vi "Open Follower Falcon.vi"(6 "Supply Current Limit Configuration":T1, 7 "refnum name":string="TalonSRX", 8 "error in (no error)":errorcluster, 9 "Master Controller to Follow":T2={"DeviceStatus"={"status"=FALSE, "code"=0, "source"=""}, "Type"=enum."PWM", "PWM"={"PWM Channel"=enum."PWM 1", "DeadBand"={"Name"="", "maxPositivePwm"=0, "minPositivePwm"=0, "centerPwm"=0, "maxNegativePwm"=0, "minNegativePwm"=0, "angularRange"=0}}, "CAN"={"Device Number"=255, "SetOutput VI Ref"=variant(enum8{"Percent VBus", "Current", "Speed", "Position", "Voltage"} enum."Percent VBus"), "GetOutput VI Ref"=variant(refnum<k1> refnum), "Enable VI Ref"=variant(dbl 12.0), "Disable VI Ref"=variant(enum8{"Percent VBus", "Speed", "Position", "Slave", "Unchanged / Invalid", "Voltage Compensation", "Current", "Motion Profile"} enum."Percent VBus"), "Data"=variant}, "Invert"=FALSE, "DIO PWM"={"PWM \"Enable\" Channel"=enum."Invalid", "DIOChannel"=enum."Invalid", "PWM Rate"=0.0}}, 10 "Invert?":bool, 11 "Device Number":u8) -> (0 "error out":errorcluster)   [LabVIEW 2019, in "Drive.lvlib" / "Falcon500.lvclass"]
uses:
  Falcon500.lvclass
  <vilib>/Rock Robotics/WPI/ThirdParty/Phoenix-LabVIEW/Motor Controller/Controls/CTRE_Phoenix_MotorControl_TalonFXInvertType.ctl
  <vilib>/Rock Robotics/SystemInterfaces/DIO/FPGA_DIOPWMChannel.ctl
  <vilib>/Rock Robotics/WPI/PWM/WPI_PWMDeadband.ctl
  <vilib>/Rock Robotics/WPI/MotorControl/WPI_MotorControlType.ctl
  <vilib>/Rock Robotics/SystemInterfaces/DIO/FPGA_DIOChannel.ctl
  <vilib>/Rock Robotics/WPI/MotorControl/WPI_MotorControlDeviceRef.ctl
  <vilib>/Rock Robotics/WPI/ThirdParty/Phoenix-LabVIEW/Motor Controller/Controls/CTRE_Phoenix_MotorControl_SupplyCurrentLimitConfiguration.ctl
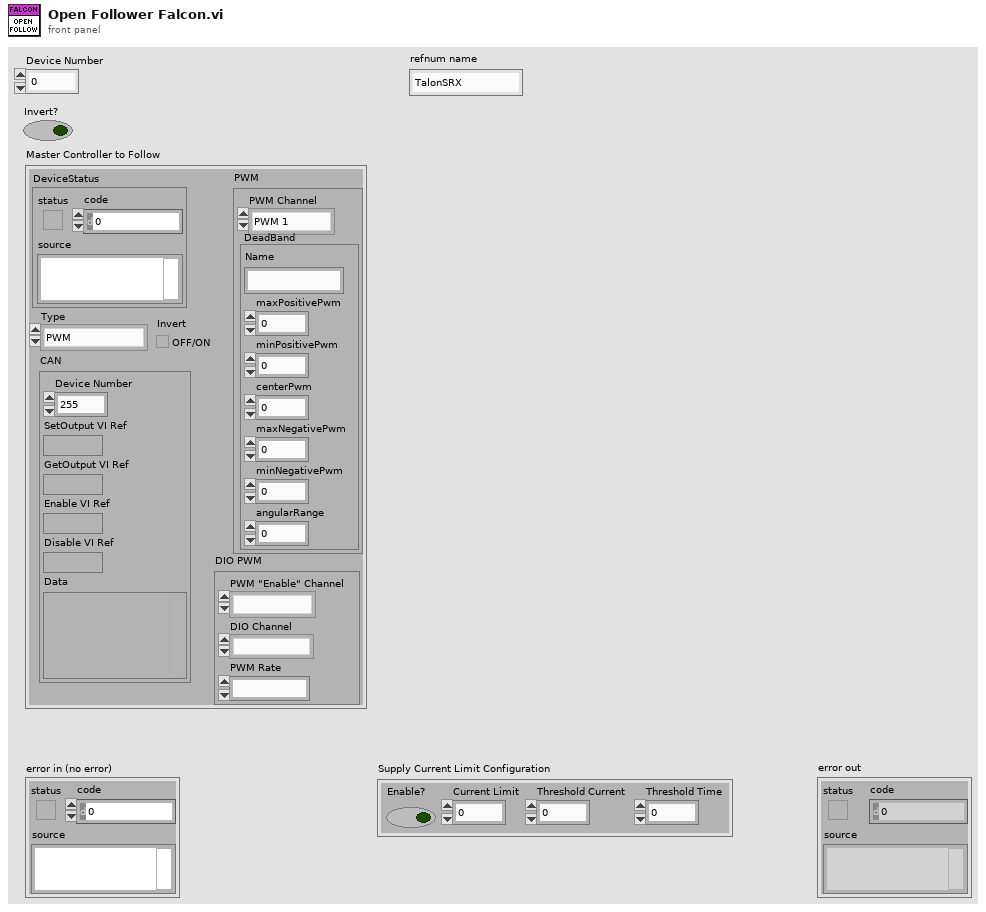
[diagram p1: front panel]
types:
  T1 = typedef "CTRE_Phoenix_MotorControl_SupplyCurrentLimitConfiguration.ctl" = cluster{"Enable?":bool, "Current Limit":dbl, "Threshold Current":dbl, "Threshold Time":dbl}
  T2 = typedef "WPI_MotorControlDeviceRef.ctl" = cluster{"DeviceStatus":errorcluster, "Type":T3, "PWM":cluster{"PWM Channel":T4, "DeadBand":T5}, "CAN":cluster{"Device Number":u8, "SetOutput VI Ref":variant, "GetOutput VI Ref":variant, "Enable VI Ref":variant, "Disable VI Ref":variant, "Data":variant}, "Invert":bool, "DIO PWM":cluster{"PWM \"Enable\" Channel":T4, "DIOChannel":T6, "PWM Rate":dbl}}
  T3 = typedef "WPI_MotorControlType.ctl" = enum16{"PWM", "CAN", "DIO PWM"}
  T4 = typedef "FPGA_DIOPWMChannel.ctl" = enum8{"PWM 0", "PWM 1", "PWM 2", "PWM 3", "PWM 4", "PWM 5", "PWM 6", "PWM 7", "PWM 8", "PWM 9", "PWM MXP 0", "PWM MXP 1", "PWM MXP 2", "PWM MXP 3", "PWM MXP 4", "PWM MXP 5", "PWM MXP 6", "PWM MXP 7", "PWM MXP 8", "PWM MXP 9", "Invalid"}
  T5 = typedef "WPI_PWMDeadband.ctl" = cluster{"Name":string, "maxPositivePwm":i32, "minPositivePwm":i32, "centerPwm":i32, "maxNegativePwm":i32, "minNegativePwm":i32, "angularRange":u16}
  T6 = typedef "FPGA_DIOChannel.ctl" = enum8{"DIO 0", "DIO 1", "DIO 2", "DIO 3", "DIO 4", "DIO 5", "DIO 6", "DIO 7", "DIO 8", "DIO 9", "DIO MXP 0", "DIO MXP 1", "DIO MXP 2", "DIO MXP 3", "DIO MXP 4", "DIO MXP 5", "DIO MXP 6", "DIO MXP 7", "DIO MXP 8", "DIO MXP 9", "DIO MXP 10", "DIO MXP 11", "DIO MXP 12", "DIO MXP 13", "DIO MXP 14", "DIO MXP 15", "SPI Port CS1", "SPI Port CS2", "SPI Port CS3", "SPI Port MISO", "SPI Port MOSI", "Invalid"}
  T7 = typedef "CTRE_Phoenix_MotorControl_TalonFXInvertType.ctl" = enum16{"Counter-Clockwise", "Clockwise"}
  T8 = enum16{"FollowerType_PercentOutput", "FollowerType_AuxOutput1"}
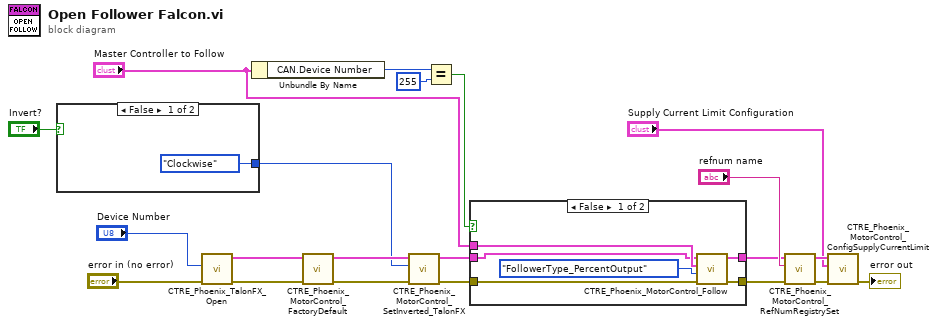
[diagram p0: block diagram]
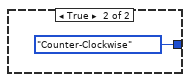
[diagram p2: hidden frame]
diagram:
  n1 = case shown="False" "Invert?" {
    tunnel: [CTRE_Phoenix_MotorControl_TalonFXInvertType."Clockwise" ("Invert Type") CTRE_Phoenix_MotorControl_TalonFXInvertType."Counter-Clockwise" ("Invert Type")] -> w7
    frame False {
    }
    frame True {
    }
  }
  n2 = call <vilib>:"CTRE_Phoenix_TalonFX_Open.vi"("error in"="error in (no error)", "Device Number"="Device Number") -> ("error out"=w17:errorcluster, "CAN Talon SRX Ref"=w16:T2)  [unwired: 8 in]
  n3 = Unbundle By Name("Master Controller to Follow") -> ("CAN.Device Number"=w14:u8)
  n4 = call <vilib>:"CTRE_Phoenix_MotorControl_FactoryDefault.vi"("error in"=w17, "PhoenixMotorControlDevRef"=w16) -> ("error out"=w10:errorcluster, "PhoenixMotorControlDevRef"=w11:T2)  [unwired: 8 in]
  n5 = call <vilib>:"CTRE_Phoenix_MotorControl_SetInverted_TalonFX.vi"("error in (no error)"=w10, "Invert Type"=w7, "PhoenixMotorControlDevRef"=w11) -> ("error out"=w9:errorcluster, "PhoenixMotorControlDevRef"=w8:T2)  [unwired: 7 in]
  n6 = Equal?(x=w14, y=u8 255) -> (x = y?=w12:bool)
  n7 = case shown="False" w12 {
    tunnel: [w29 w30] -> w20
    tunnel: [w28 w31] -> w19
    tunnel: w9 -> [w27 w30]
    tunnel: "Master Controller to Follow" -> [w26 _]
    tunnel: w8 -> [w25 w31]
    frame False {
      n8 = call <vilib>:"CTRE_Phoenix_MotorControl_Follow.vi"("error in (no error)"=w27, "FollowerType"=T8."FollowerType_PercentOutput", "Master Controller to Follow"=w26, "PhoenixMotorControlDevRef"=w25) -> ("error out"=w29:errorcluster, "PhoenixMotorControlDevRef"=w28:T2)  [unwired: 6 in]
    }
    frame True {
    }
  }
  n9 = call <vilib>:"CTRE_Phoenix_MotorControl_RefNumRegistrySet.vi"("error in (no error)"=w20, "refnum name"="refnum name", "PhoenixMotorControlDevRef"=w19) -> ("error out"=w6:errorcluster, "PhoenixMotorControlDevRef"=w4:T2)  [unwired: 7 in]
  n10 = call <vilib>:"CTRE_Phoenix_MotorControl_ConfigSupplyCurrentLimit.vi"("error in (no error)"=w6, "Supply Current Limit Configuration"="Supply Current Limit Configuration", "PhoenixMotorControlDevRef"=w4) -> ("error out"=→"error out":errorcluster)  [unwired: 7 in, 1 out]
